vi "sub_run actuators.vi"(0 "Actuator Task":refnum<k21>, 5 "Actuator error":errorcluster, 7 "Inputs":dbl[][](array[numeric]), 11 "T_control":dbl[](array[numeric]), 12 "Iteration":i32, 13 "Control Counter in":i32) -> (4 "task out":refnum<k21>, 6 "error out":errorcluster, 15 "Control Counter out":i32)   [LabVIEW 2020]
uses:
  <vilib>/DAQmx/write.llb/DAQmx Write (Analog 1D DBL NChan 1Samp).vi
  globalvariables.vi
  <vilib>/addons/control/pid/pid.llb/PID (DBL Array).vi
  <vilib>/DAQmx/miscellaneous.llb/DAQmx Fill In Error Info.vi
  <vilib>/addons/control/pid/NI_PID_pid.lvlib
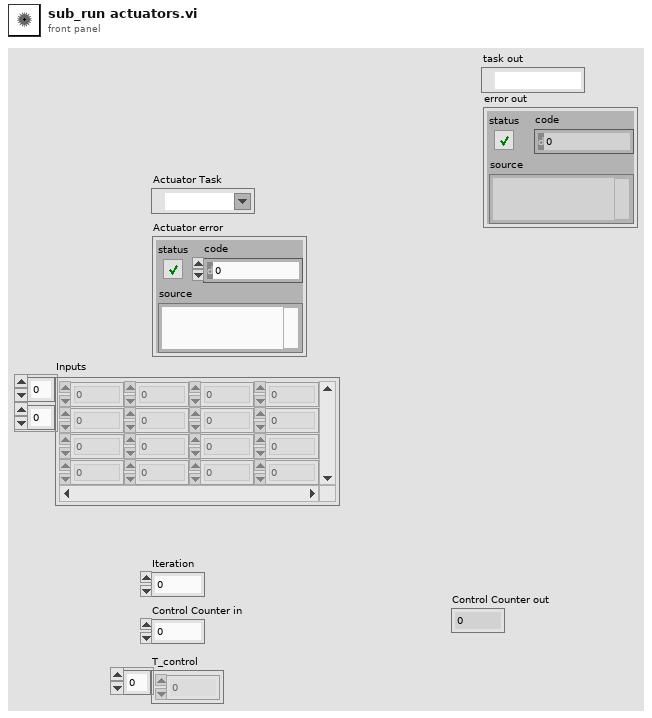
[diagram p1: front panel]
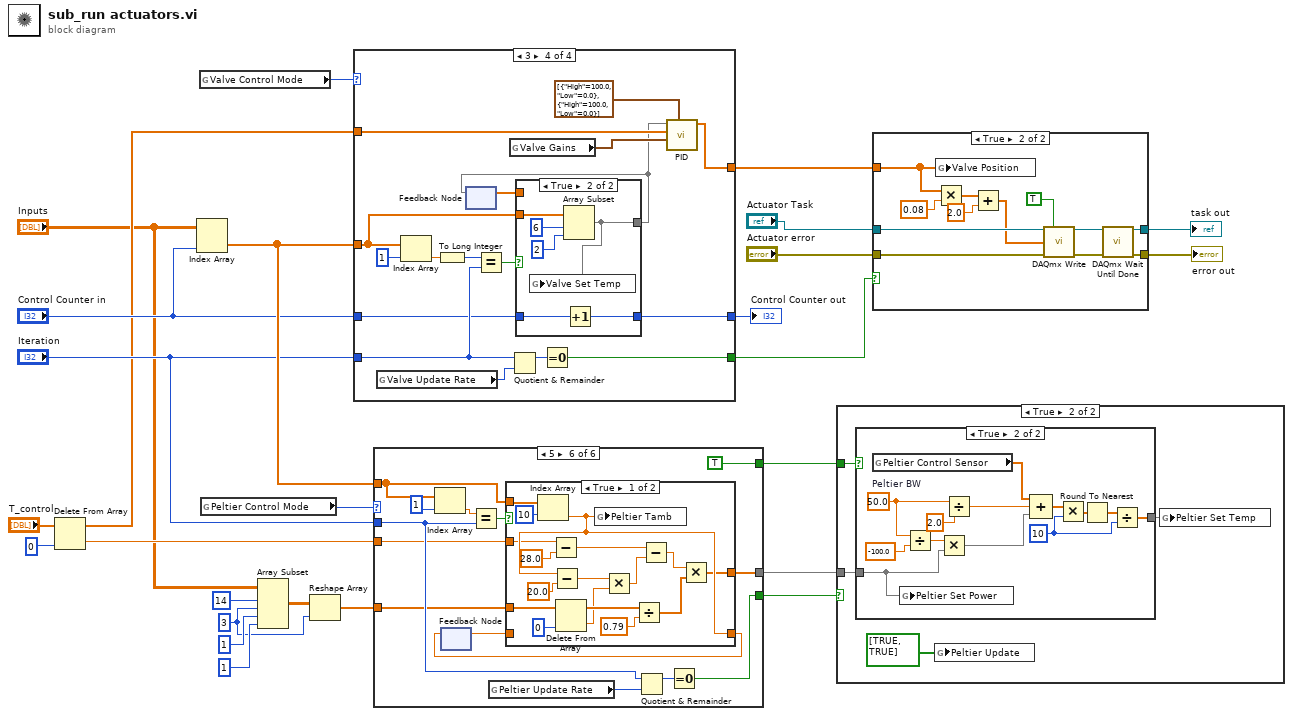
[diagram p0: block diagram]
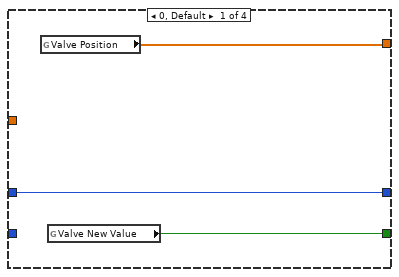
[diagram p4: hidden frame]
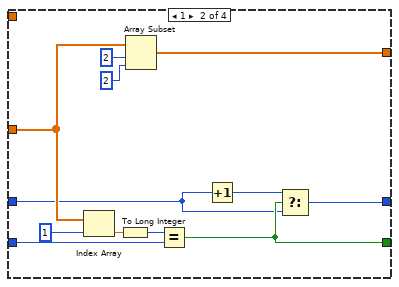
[diagram p5: hidden frame]
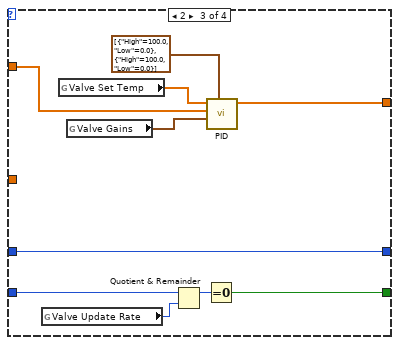
[diagram p6: hidden frame]
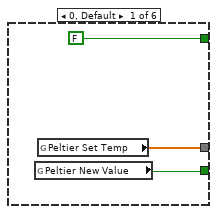
[diagram p9: hidden frame]
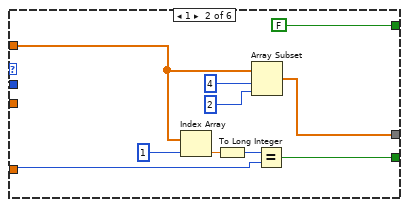
[diagram p10: hidden frame]
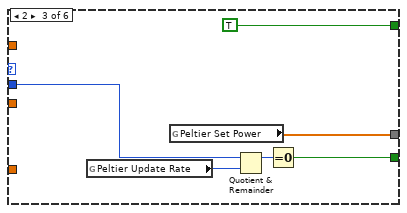
[diagram p11: hidden frame]
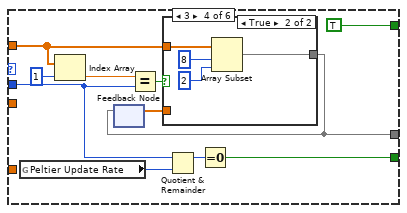
[diagram p12: hidden frame]
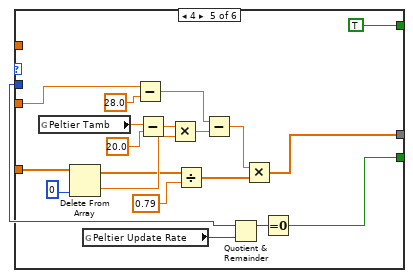
[diagram p14: hidden frame]
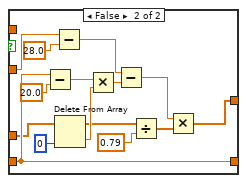
[diagram p15: hidden frame]
diagram:
  w2 = 3 ("length")
  n1 = Delete From Array(array="T_control", index=0 ("length")) -> (deleted portion=w9:dbl, array with subset deleted=w8:dbl[])  [unwired: 1 in]
  n2 = Index Array(array="Inputs", index (col)="Control Counter in") -> (element=w20:dbl[])  [unwired: 1 in]
  n3 = global read "globalvariables.vi" "Valve Control Mode"() -> (w21:i16)
  n4 = global read "globalvariables.vi" "Peltier Control Mode"() -> (w26:i16)
  n5 = Array Subset(array="Inputs", index (row)=14 ("index"), length (row)=w2, index (col)=1 ("index"), length (col)=1 ("length")) -> (w3:dbl[][])
  n6 = Reshape Array(w3, w2) -> (w1:dbl[])
  n7 = case shown="3" w21 {
    tunnel: w20 -> [_ w35 _ w60]
    tunnel: [w28 w33 w48 w67] -> w19
    tunnel: [w29 w41 w43 w52] -> w18
    tunnel: "Iteration" -> [_ w34 w49 w62]
    tunnel: w8 -> [_ _ w44 w54]
    tunnel: [w27 w32 w42 w59] -> w16
    tunnel: "Control Counter in" -> [w27 w30 w42 w58]
    frame 0, Default {
      n8 = global read "globalvariables.vi" "Valve Position"() -> (w29:dbl[])
      n9 = global read "globalvariables.vi" "Valve New Value"() -> (w28:bool)
    }
    frame 1 {
      n10 = Index Array(array=w35, index=1 ("index (row)")) -> (element=w37:dbl)
      n11 = To Long Integer(number=w37) -> (32bit integer=w36:i32)
      n12 = Array Subset(array=w35, index=2, length=2) -> (w41:dbl[])
      n13 = Equal?(x=w36, y=w34) -> (x = y?=w33:bool)
      n14 = Increment(x=w30) -> (x+1=w31:i32)
      n15 = Select(t=w31, s=w33, f=w30) -> (s? t:f=w32:i32)
    }
    frame 2 {
      n16 = global read "globalvariables.vi" "Valve Update Rate"() -> (w51:i32)
      n17 = global read "globalvariables.vi" "Valve Set Temp"() -> (w46:dbl[])
      n18 = global read "globalvariables.vi" "Valve Gains"() -> (w45:cluster{"P":dbl, "I":dbl, "D":dbl}[])
      n19 = Quotient & Remainder(x=w49, y=w51) -> (x-y*floor(x/y)=w50:i32)  [unwired: 1 out]
      n20 = Equal To 0?(x=w50) -> (x = 0?=w48:bool)
      n21 = call-poly <vilib>:"PID.vi"("output range"=cluster{"High":dbl, "Low":dbl}[] [{"High"=100.0, "Low"=0.0}, {"High"=100.0, "Low"=0.0}], "PID gains"=w45, "process variable"=w44, "setpoint"=w46) -> ("output"=w43:dbl[])  [unwired: 6 in, 1 out]
    }
    frame 3 {
      n22 = global read "globalvariables.vi" "Valve Update Rate"() -> (w68:i32)
      n23 = Index Array(array=w60, index=1 ("index (row)")) -> (element=w65:dbl)
      n24 = To Long Integer(number=w65) -> (32bit integer=w64:i32)
      n25 = feedback #1() -> (w57:dbl[])  [unwired: 1 in]
      n26 = Equal?(x=w64, y=w62) -> (x = y?=w61:bool)
      n27 = global read "globalvariables.vi" "Valve Gains"() -> (w56:cluster{"P":dbl, "I":dbl, "D":dbl}[])
      n28 = Quotient & Remainder(x=w62, y=w68) -> (x-y*floor(x/y)=w66:i32)  [unwired: 1 out]
      n29 = case shown="True" w61 {
        tunnel: w60 -> [_ w76]
        tunnel: [w70 w71] -> w53
        tunnel: w57 -> [w70 _]
        tunnel: [w69 w73] -> w59
        tunnel: w58 -> [w69 w74]
        frame False {
        }
        frame True {
          n30 = Array Subset(array=w76, index=6 ("index (row)"), length=2) -> (w71:dbl[])
          n31 = global write "globalvariables.vi" "Valve Set Temp"(w71) -> ()
          n32 = Increment(x=w74) -> (x+1=w73:i32)
        }
      }
      n33 = feedback-in #1(w53) -> ()
      n34 = Equal To 0?(x=w66) -> (x = 0?=w67:bool)
      n35 = call-poly <vilib>:"PID.vi"("output range"=cluster{"High":dbl, "Low":dbl}[] [{"High"=100.0, "Low"=0.0}, {"High"=100.0, "Low"=0.0}], "PID gains"=w56, "process variable"=w54, "setpoint"=w53) -> ("output"=w52:dbl[])  [unwired: 6 in, 1 out]
    }
  }
  "Control Counter out" <- w16
  n36 = case shown="5" w26 {
    tunnel: w20 -> [_ w84 _ w99 _ w138]
    tunnel: "Iteration" -> [_ w85 w93 w100 w128 w139]
    tunnel: [w79 w86 w92 w103 w129 w142] -> w14
    tunnel: w9 -> [_ _ _ _ w119 w136]
    tunnel: [w78 w81 w91 w98 w116 w135] -> w13
    tunnel: [FALSE FALSE TRUE TRUE TRUE TRUE] -> w12
    tunnel: w1 -> [_ _ _ _ w117 w133]
    frame 0, Default {
      n37 = global read "globalvariables.vi" "Peltier New Value"() -> (w79:bool)
      n38 = global read "globalvariables.vi" "Peltier Set Temp"() -> (w78:dbl[])
    }
    frame 1 {
      n39 = Index Array(array=w84, index=1 ("index (row)")) -> (element=w88:dbl)
      n40 = To Long Integer(number=w88) -> (32bit integer=w87:i32)
      n41 = Array Subset(array=w84, index=4 ("index (row)"), length=2) -> (w81:dbl[])
      n42 = Equal?(x=w87, y=w85) -> (x = y?=w86:bool)
    }
    frame 2 {
      n43 = global read "globalvariables.vi" "Peltier Update Rate"() -> (w94:i32)
      n44 = global read "globalvariables.vi" "Peltier Set Power"() -> (w91:dbl[])
      n45 = Quotient & Remainder(x=w93, y=w94) -> (x-y*floor(x/y)=w95:i32)  [unwired: 1 out]
      n46 = Equal To 0?(x=w95) -> (x = 0?=w92:bool)
    }
    frame 3 {
      n47 = global read "globalvariables.vi" "Peltier Update Rate"() -> (w105:i32)
      n48 = Index Array(array=w99, index=1 ("index (row)")) -> (element=w96:dbl)
      n49 = feedback #2() -> (w104:dbl[])  [unwired: 1 in]
      n50 = Equal?(x=w96, y=w100) -> (x = y?=w101:bool)
      n51 = case shown="True" w101 {
        tunnel: w99 -> [_ w110]
        tunnel: [w107 w108] -> w98
        tunnel: w104 -> [w107 _]
        frame False {
        }
        frame True {
          n52 = Array Subset(array=w110, index=8 ("index (row)"), length=2) -> (w108:dbl[])
        }
      }
      n53 = feedback-in #2(w98) -> ()
      n54 = Quotient & Remainder(x=w100, y=w105) -> (x-y*floor(x/y)=w106:i32)  [unwired: 1 out]
      n55 = Equal To 0?(x=w106) -> (x = 0?=w103:bool)
    }
    frame 4 {
      n56 = global read "globalvariables.vi" "Peltier Tamb"() -> (w118:dbl)
      n57 = Delete From Array(array=w117, index=0 ("length")) -> (deleted portion=w125:dbl, array with subset deleted=w112:dbl[])  [unwired: 1 in]
      n58 = global read "globalvariables.vi" "Peltier Update Rate"() -> (w130:i32)
      n59 = Subtract(x=w119, y=28.0) -> (x-y=w126:dbl)
      n60 = Subtract(x=w118, y=20.0) -> (x-y=w114:dbl)
      n61 = Multiply(x=w114, y=w125) -> (x*y=w115:dbl)
      n62 = Divide(x=w112, y=0.79) -> (x/y=w124:dbl[])
      n63 = Subtract(x=w126, y=w115) -> (x-y=w113:dbl)
      n64 = Quotient & Remainder(x=w128, y=w130) -> (x-y*floor(x/y)=w131:i32)  [unwired: 1 out]
      n65 = Multiply(x=w113, y=w124) -> (x*y=w116:dbl[])
      n66 = Equal To 0?(x=w131) -> (x = 0?=w129:bool)
    }
    frame 5 {
      n67 = Index Array(array=w138, index=1 ("index (row)")) -> (element=w132:dbl)
      n68 = feedback #3() -> (w143:dbl)  [unwired: 1 in]
      n69 = Equal?(x=w132, y=w139) -> (x = y?=w140:bool)
      n70 = global read "globalvariables.vi" "Peltier Update Rate"() -> (w144:i32)
      n71 = case shown="True" w140 {
        tunnel: w138 -> [w162 _]
        tunnel: [w148 w177] -> w135
        tunnel: w143 -> [_ w174]
        tunnel: [w153 w174] -> w137
        tunnel: w136 -> [w152 w176]
        tunnel: w133 -> [w154 w170]
        frame True {
          n72 = Index Array(array=w162, index=10 ("index (row)")) -> (element=w153:dbl)
          n73 = Subtract(x=w152, y=28.0) -> (x-y=w158:dbl)
          n74 = Subtract(x=w153, y=20.0) -> (x-y=w149:dbl)
          n75 = Delete From Array(array=w154, index=0 ("length")) -> (deleted portion=w159:dbl, array with subset deleted=w160:dbl[])  [unwired: 1 in]
          n76 = global write "globalvariables.vi" "Peltier Tamb"(w153) -> ()
          n77 = Multiply(x=w149, y=w159) -> (x*y=w150:dbl)
          n78 = Divide(x=w160, y=0.79) -> (x/y=w146:dbl[])
          n79 = Subtract(x=w158, y=w150) -> (x-y=w151:dbl)
          n80 = Multiply(x=w151, y=w146) -> (x*y=w148:dbl[])
        }
        frame False {
          n81 = Subtract(x=w174, y=20.0) -> (x-y=w167:dbl)
          n82 = Subtract(x=w176, y=28.0) -> (x-y=w172:dbl)
          n83 = Delete From Array(array=w170, index=0 ("length")) -> (deleted portion=w169:dbl, array with subset deleted=w168:dbl[])  [unwired: 1 in]
          n84 = Multiply(x=w167, y=w169) -> (x*y=w166:dbl)
          n85 = Subtract(x=w172, y=w166) -> (x-y=w165:dbl)
          n86 = Divide(x=w168, y=0.79) -> (x/y=w163:dbl[])
          n87 = Multiply(x=w165, y=w163) -> (x*y=w177:dbl[])
        }
      }
      n88 = feedback-in #3(w137) -> ()
      n89 = Quotient & Remainder(x=w139, y=w144) -> (x-y*floor(x/y)=w145:i32)  [unwired: 1 out]
      n90 = Equal To 0?(x=w145) -> (x = 0?=w142:bool)
    }
  }
  n91 = case shown="True" w14 {
    tunnel: w13 -> [_ w180]
    tunnel: w12 -> [_ w179]
    frame False {
    }
    frame True {
      n92 = case shown="True" w179 {
        tunnel: w180 -> [w182 w188]
        tunnel: [w182 w183] -> w178
        frame False {
        }
        frame True {
          w186 = 10
          w191 = 50.0  # Peltier BW
          n93 = global read "globalvariables.vi" "Peltier Control Sensor"() -> (w195:dbl[])
          n94 = global write "globalvariables.vi" "Peltier Set Power"(w188) -> ()
          n95 = Divide(x=w191, y=-100.0) -> (x/y=w194:dbl)
          n96 = Multiply(x=w194, y=w188) -> (x*y=w189:dbl[])
          n97 = Divide(x=w191, y=2.0) -> (x/y=w193:dbl)
          n98 = Compound Arithmetic op=ADD(w195, w193, w189) -> (w184:dbl[])
          n99 = Multiply(x=w184, y=w186) -> (x*y=w185:dbl[])
          n100 = Round To Nearest(number=w185) -> (nearest integer value=w187:dbl[])
          n101 = Divide(x=w187, y=w186) -> (x/y=w183:dbl[])
        }
      }
      n102 = global write "globalvariables.vi" "Peltier Update"(bool[] [TRUE, TRUE]) -> ()
      n103 = global write "globalvariables.vi" "Peltier Set Temp"(w178) -> ()
    }
  }
  n104 = case shown="True" w19 {
    tunnel: [w197 w206] -> w25
    tunnel: [w196 w205] -> w24
    tunnel: "Actuator Task" -> [w197 w204]
    tunnel: "Actuator error" -> [w196 w203]
    tunnel: w18 -> [_ w198]
    frame False {
    }
    frame True {
      n105 = global write "globalvariables.vi" "Valve Position"(w198) -> ()
      n106 = Multiply(x=w198, y=0.08) -> (x*y=w202:dbl[])
      n107 = Add(x=w202, y=2.0 ("x")) -> (x+y=w199:dbl[])
      n108 = call-poly <vilib>:"DAQmx Write.vi"("task/channels in"=w204, "auto start"=TRUE, "data"=w199, "error in"=w203) -> ("task out"=w208:refnum<k21>, "error out"=w209:errorcluster)  [unwired: 9 in, 1 out]
      n109 = call <vilib>:"DAQmx Wait Until Done.vi"("task/channels in"=w208, "error in"=w209) -> ("task out"=w206:refnum<k21>, "error out"=w205:errorcluster)  [unwired: 12 in]
    }
  }
  "task out" <- w25
  "error out" <- w24
